vi "U16.vi"(1 "Numeric Input":u16) -> (0 "Numeric Output":u16)   [LabVIEW 2011]
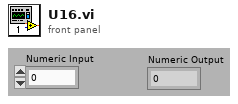
[diagram p1: front panel]
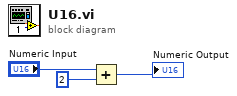
[diagram p0: block diagram]
diagram:
  n1 = Add(x="Numeric Input", y=u16 2) -> (x+y=→"Numeric Output":u16)
